vi "DAC_manual_ramp.vi"() -> ()   [LabVIEW 2013]
uses:
  <vilib>/DAQmx/read.llb/DAQmx Read (Analog 2D DBL NChan NSamp).vi
  <vilib>/DAQmx/create/channels.llb/DAQmx Create Channel (AI-Voltage-Basic).vi
  <vilib>/DAQmx/miscellaneous.llb/DAQmx Fill In Error Info.vi
  <resource>/objmgr/daqmx.rc
panel:
  out "Imin":dbl
  out "R":dbl
  in  "Back to\ninit value":bool
  in  "ADC Gain":u32(ring)=1 items=["1e6"=1000, "1e7"=100, "1e8"=10, "1e9"=1]
  in  "Save data":bool
  out "Ydata":dbl[][](array[numeric])
  out "Xdata":dbl[][](array[numeric])
  out "ADC values":dbl[](array[numeric])
  in  "DAC param":T1={"IP Adress FPGA"="192.168.137.11", "Delay(us)"=100, "Busses to use"=[TRUE, TRUE, TRUE, TRUE, TRUE, FALSE, FALSE, FALSE], "max"=0.5, "min"=-2.0}
  in  "Clear graph":bool
  in  "ADC channel":dbl
  in  "Stop":bool
  in  "Go":bool
  in  "time per pt (ms)":dbl=100.0
  in  "Xparam":dbl
  out "XY Graph":cluster{dbl[], dbl[]}(graph)
  in  "Nb of points":u32=101
  in  "Ramps":T2(array[cluster]) {"index" items=["0", "1", "2", "3", "4", "5", "6", "7"]; "bus" items=["0", "1", "2", "3", "4", "5", "6", "7"]}
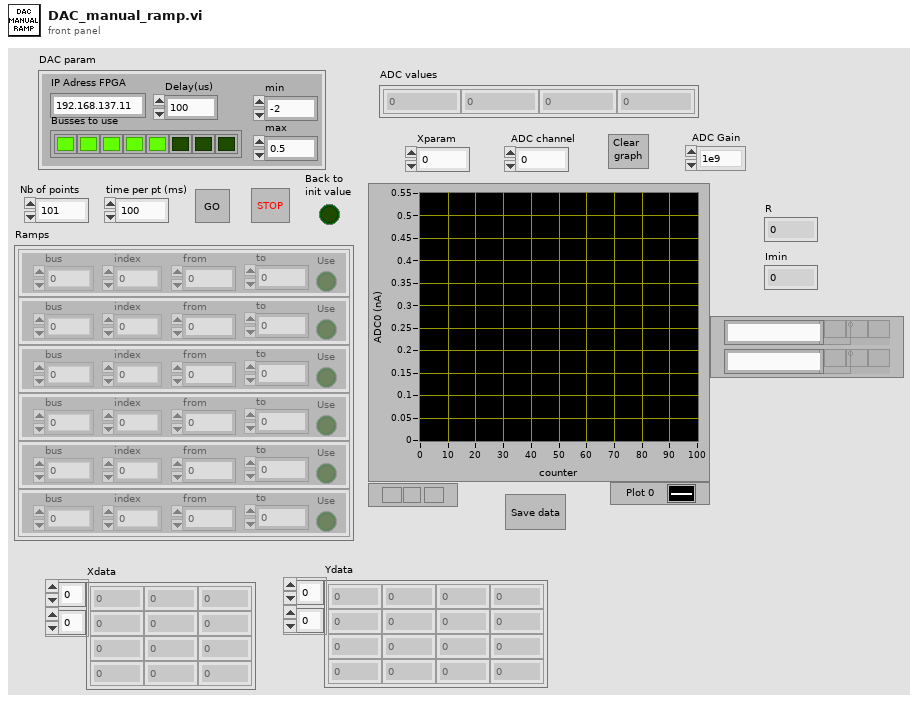
[diagram p1: front panel]
types:
  T1 = cluster{"IP Adress FPGA":string, "Delay(us)":u8, "Busses to use":bool[], "max":dbl, "min":dbl}
  T2 = cluster{"bus":u16, "index":u16, "from":dbl, "to":dbl, "Use":bool}[]
  T3 = enum8{"start movement", "buses to use", "delay", "value", "stop", ""}
  T4 = cluster{"bus":u16, "index":u16, "from":dbl, "to":dbl, "Use":bool}
  T5 = typedef "fpga-bitfile-ref.ctl" = refnum<k20>
  T6 = enum8{"start movement", "buses to use", "delay", "value"}
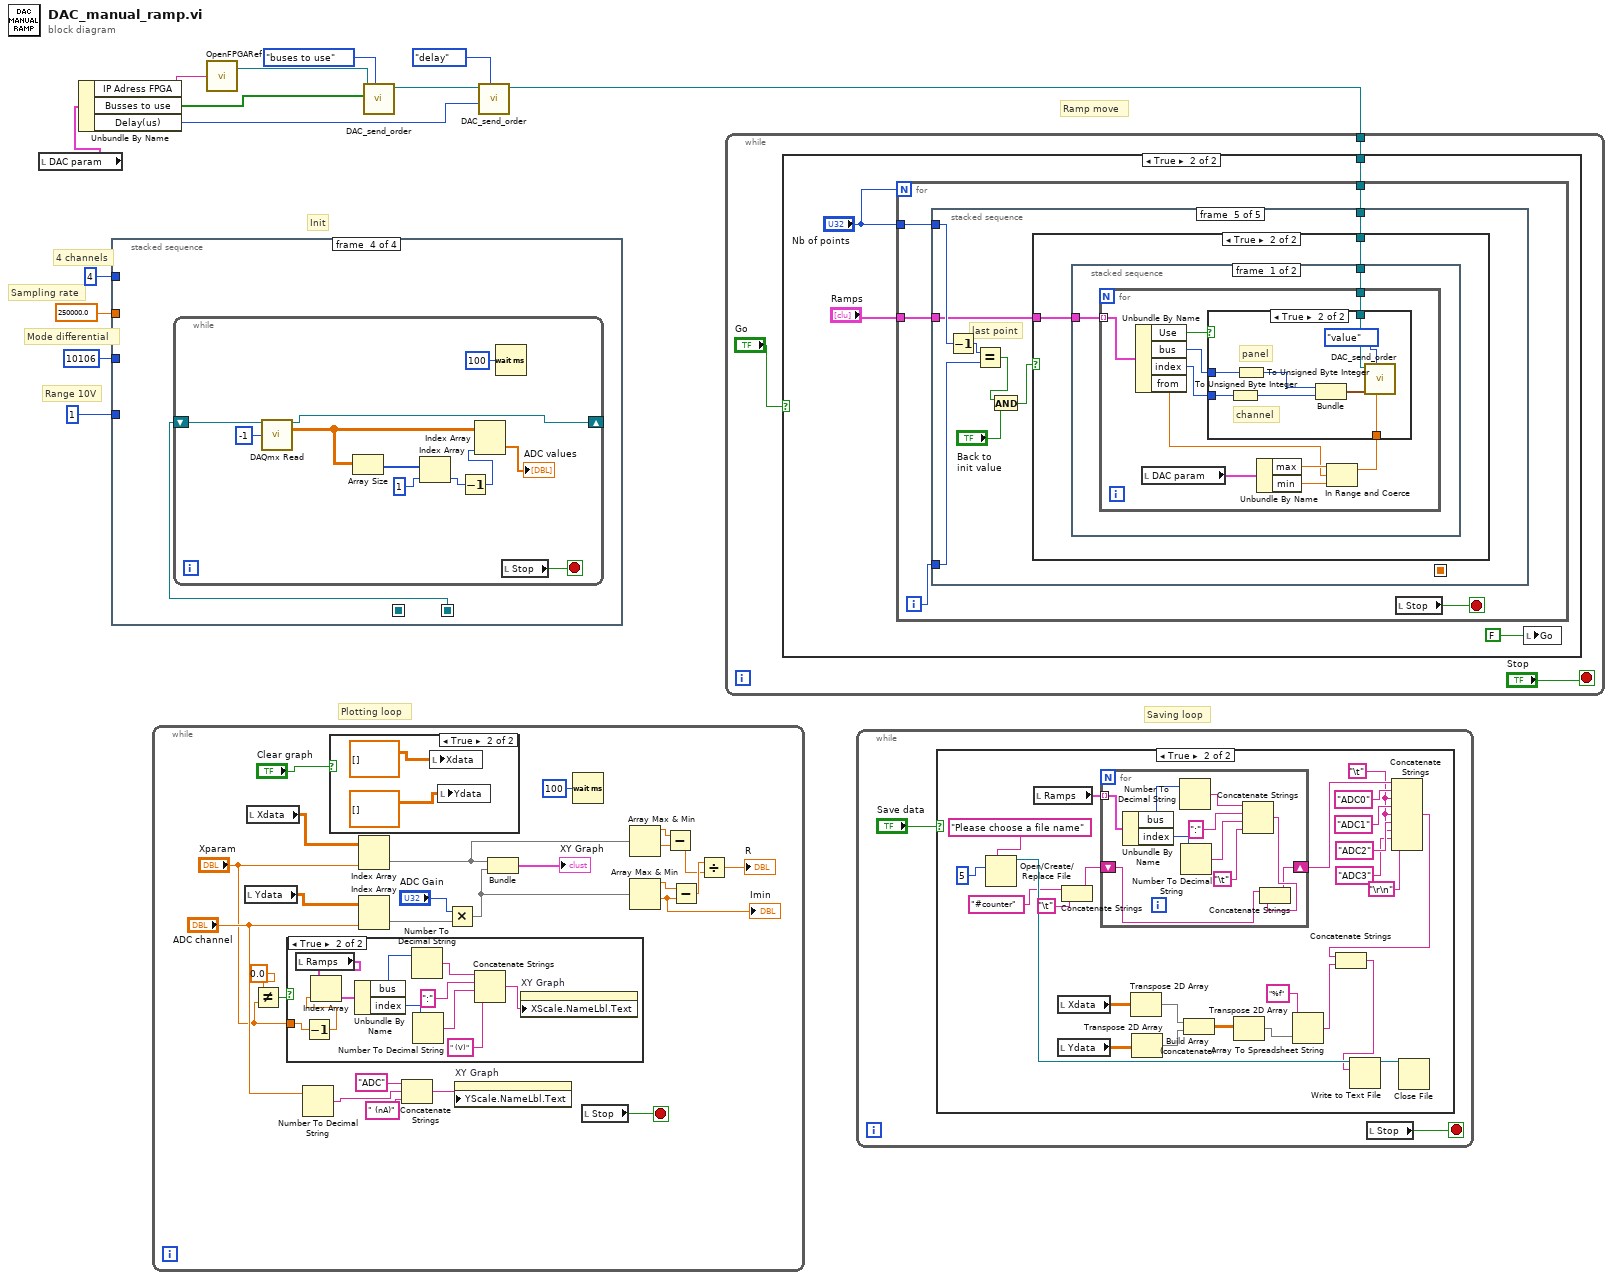
[diagram p0: block diagram]
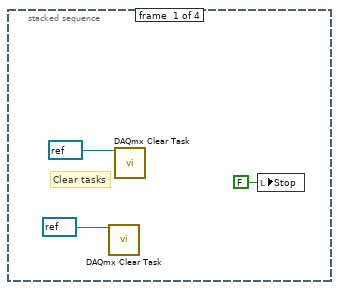
[diagram p2: hidden frame]
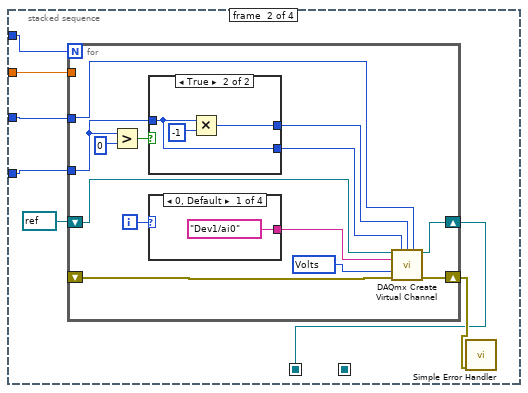
[diagram p3: hidden frame]
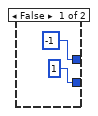
[diagram p4: hidden frame]
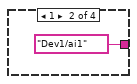
[diagram p5: hidden frame]
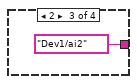
[diagram p6: hidden frame]
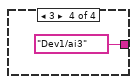
[diagram p7: hidden frame]
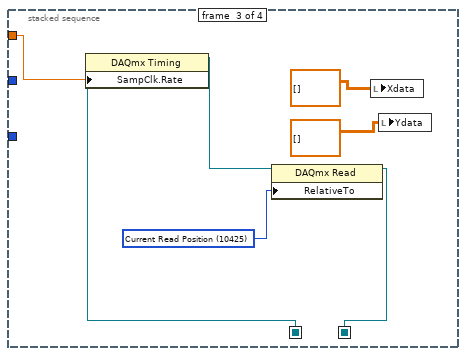
[diagram p8: hidden frame]
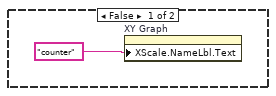
[diagram p10: hidden frame]
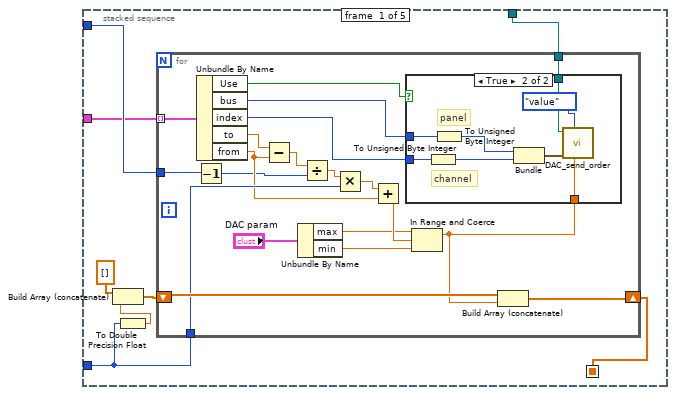
[diagram p12: hidden frame]
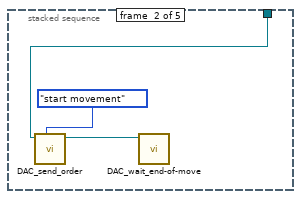
[diagram p14: hidden frame]
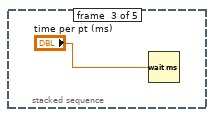
[diagram p15: hidden frame]
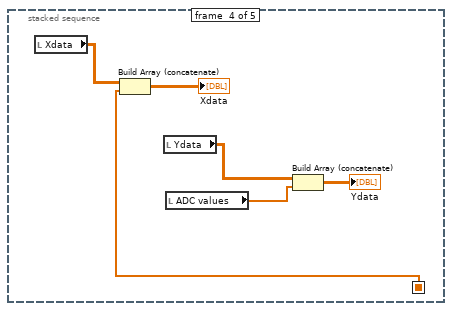
[diagram p16: hidden frame]
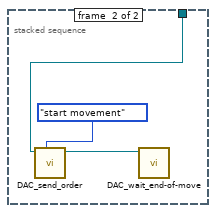
[diagram p19: hidden frame]
diagram:
  # "Init"
  # "Sampling rate"
  # "Mode differential"
  # "Range 10V"
  # "4 channels"
  # "Plotting loop"
  # "Ramp move"
  # "Saving loop"
  n1 = local read "DAC param"() -> (w6:T1)
  n2 = Unbundle By Name(w6) -> ("IP Adress FPGA"=w9:string, "Busses to use"=w8:bool[], "Delay(us)"=w7:u8)
  n3 = stacked-sequence {
    seq-local: [_ w17 _ _] -> [_ _ w51 _]
    seq-local: [_ _ w48 _] -> [_ _ _ w53]
    tunnel: 4 -> [_ w22 _ _]
    tunnel: 10106 -> [_ w21 _ _]
    tunnel: 1 -> [_ w20 _ _]
    tunnel: 250000.0 -> [_ w19 w52 _]
    frame #0 {
      # "Clear tasks"
      n4 = call <vilib>:"DAQmx Clear Task.vi"("task in"=refnum<k21> refnum ("task out in")) -> ()  [unwired: 14 in, 1 out]
      n5 = call <vilib>:"DAQmx Clear Task.vi"("task in"=refnum<k21> refnum ("task out in")) -> ()  [unwired: 14 in, 1 out]
      n6 = local write "Stop"(FALSE ("Stop")) -> ()
    }
    frame #1 {
      n7 = for {
        N: w22 -> [_]
        shift-right: [w24] -> w17
        shift-left: refnum<k21> refnum ("task out") -> [w36]
        shift-right: [w33] -> w23
        shift-left: _ -> [w25]
        tunnel: w20 -> [w30]
        tunnel: w21 -> [w26]
        tunnel: w19 -> [_]
        i -> [w27]
        w34 = 10348 items=["Volts"=10348, "From Custom Scale"=10065] ("units")
        n8 = Greater?(x=w30, y=i16 0) -> (0:w31:bool)
        n9 = case shown="True" w31 {
          tunnel: w30 -> [_ w39]
          tunnel: [i16 -1 w40] -> w32
          tunnel: [i16 1 ("Range") w39] -> w28
          frame False {
          }
          frame True {
            n10 = Multiply(x=w39, y=i16 -1) -> (x*y=w40:i32)
          }
        }
        n11 = case shown="0, Default" w27 {
          tunnel: [tag "Dev1/ai0" ("physical channels") tag "Dev1/ai1" ("physical channels") tag "Dev1/ai2" ("physical channels") tag "Dev1/ai3" ("physical channels")] -> w35
          frame 0, Default {
          }
          frame 1 {
          }
          frame 2 {
          }
          frame 3 {
          }
        }
        n12 = call-poly <vilib>:"DAQmx Create Virtual Channel.vi"("task in"=w36, "maximum value"=w28, "minimum value"=w32, "input terminal configuration"=w26, "physical channels"=w35, "units"=w34, "error in"=w25) -> ("task out"=w24:refnum<k21>, "error out"=w33:errorcluster)  [unwired: 2 in, 5 out]
      }
      n13 = call <vilib>:"Simple Error Handler.vi"("error in (no error)"=w23) -> ()  [unwired: 4 in, 5 out]
    }
    frame #2 {
      w50 = 10425 items=["First Sample"=10424, "Current Read Position"=10425, "Reference Trigger"=10426, "First Pretrigger Sample"=10427, "Most Recent Sample"=10428] ("RelativeTo")
      n14 = property class="DAQmx Timing"(reference=w51, "SampClk.Rate"=w52) -> (reference out=w49:refnum<k21>)  [unwired: 1 in, 1 out]
      n15 = property class="DAQmx Read"(reference=w49, "RelativeTo"=w50) -> (reference out=w48:refnum<k21>)  [unwired: 1 in, 1 out]
      n16 = local write "Xdata"(dbl[][] []) -> ()
      n17 = local write "Ydata"(dbl[][] []) -> ()
    }
    frame #3 {
      n18 = while {
        shift-right: [w58] -> _
        shift-left: w53 -> [w59]
        stop <- w64 stop-if-true
        n19 = call-poly <vilib>:"DAQmx Read.vi"("task/channels in"=w59, "number of samples per channel"=-1) -> ("task out"=w58:refnum<k21>, "data"=w61:dbl[][])  [unwired: 11 in, 1 out]
        n20 = Array Size(array=w61) -> (size(s)=w62:i32[])
        n21 = Index Array(array=w62, index=1) -> (element=w56:i32)
        n22 = Decrement(x=w56) -> (x-1=w55:i32)
        n23 = Index Array(array=w61, index (col)=w55) -> (element=→"ADC values":dbl[])  [unwired: 1 in]
        n24 = Wait (ms)(milliseconds to wait=100) -> ()  [unwired: 1 out]
        n25 = local read "Stop"() -> (w64:bool)
      }
    }
  }
  n26 = while {
    stop <- w89 stop-if-true
    n27 = local read "Ydata"() -> (w87:dbl[][])
    n28 = local read "Xdata"() -> (w88:dbl[][])
    n29 = Not Equal?(x=0.0, y="Xparam") -> (x != y?=w79:bool)
    n30 = case shown="True" w79 {
      tunnel: "Xparam" -> [_ w94]
      frame False {
        n31 = property on="XY Graph" class="XYGraph (strict)"("XScale.NameLbl.Text"="counter") -> ()  [unwired: 2 in, 2 out]
      }
      frame True {
        n32 = local read "Ramps"() -> (w103:T2)
        n33 = Decrement(x=w94) -> (x-1=w93:dbl)
        n34 = Index Array(array=w103, index=w93) -> (element=w102:T4)
        n35 = Unbundle By Name(w102) -> ("bus"=w101:u16, "index"=w100:u16)
        n36 = Number To Decimal String(number=w101) -> (decimal integer string=w98:string)  [unwired: 1 in]
        n37 = Number To Decimal String(number=w100) -> (decimal integer string=w99:string)  [unwired: 1 in]
        n38 = Concatenate Strings(w98, ":", w99, " (V)") -> (w95:string)
        n39 = property on="XY Graph" class="XYGraph (strict)"("XScale.NameLbl.Text"=w95) -> ()  [unwired: 2 in, 2 out]
      }
    }
    n40 = Number To Decimal String(number="ADC channel") -> (decimal integer string=w81:string)  [unwired: 1 in]
    n41 = case shown="True" "Clear graph" {
      frame False {
      }
      frame True {
        n42 = local write "Xdata"(dbl[][] []) -> ()
        n43 = local write "Ydata"(dbl[][] []) -> ()
      }
    }
    n44 = Index Array(array=w88, index (col)="Xparam") -> (element=w75:dbl[])  [unwired: 1 in]
    n45 = Index Array(array=w87, index (col)="ADC channel") -> (element=w71:dbl[])  [unwired: 1 in]
    n46 = Concatenate Strings("ADC", w81, " (nA)") -> (w82:string)
    n47 = Multiply(x="ADC Gain", y=w71) -> (x*y=w66:dbl[])
    n48 = property on="XY Graph" class="XYGraph (strict)"("YScale.NameLbl.Text"=w82) -> ()  [unwired: 2 in, 2 out]
    n49 = Bundle("Xdata"=w75, w66) -> (→"XY Graph":cluster{"Xdata":dbl[], dbl[]})  [unwired: 1 in]
    n50 = Wait (ms)(milliseconds to wait=100) -> ()  [unwired: 1 out]
    n51 = local read "Stop"() -> (w89:bool)
    n52 = Array Max & Min(array=w75) -> (max value=w74:dbl, min value=w73:dbl)  [unwired: 2 out]
    n53 = Array Max & Min(array=w66) -> (max value=w72:dbl, min value=w65:dbl)  [unwired: 2 out]
    "Imin" <- w65
    n54 = Subtract(x=w74, y=w73) -> (x-y=w68:dbl)
    n55 = Subtract(x=w72, y=w65) -> (x-y=w69:dbl)
    n56 = Divide(x=w69, y=w68) -> (x/y=→"R":dbl)
  }
  n57 = call "OpenFPGARef.vi"("IP Address"=w9) -> ("FPGA VI Reference Out"=w10:T5)  [unwired: 1 out]
  n58 = call "DAC_send_order.vi"("order"=T3."buses to use", "buses to use"=w8, "FPGA VI Reference In"=w10) -> ("FPGA VI Reference Out"=w11:T5)  [unwired: 8 in]
  n59 = call "DAC_send_order.vi"("order"=T3."delay", "delay between steps (us)"=w7, "FPGA VI Reference In"=w11) -> ("FPGA VI Reference Out"=w5:T5)  [unwired: 8 in]
  n60 = while {
    tunnel: w5 -> [w105]
    stop <- "Stop" stop-if-true
    n61 = case shown="True" "Go" {
      tunnel: w105 -> [_ w110]
      frame False {
      }
      frame True {
        n62 = for {
          N: "Nb of points" -> [_]
          tunnel: "Nb of points" -> [w115]
          tunnel: w110 -> [w114]
          tunnel: "Ramps" -> [w111]
          i -> [w113]
          stop <- w112 stop-if-true
          n63 = stacked-sequence {
            seq-local: [w121 _ _ _ _] -> [_ _ _ w161 _]
            tunnel: w115 -> [w123 _ _ _ w169]
            tunnel: w114 -> [w122 w154 _ _ w166]
            tunnel: w113 -> [w120 _ _ _ w165]
            tunnel: w111 -> [w116 _ _ _ w167]
            frame #0 {
              n64 = To Double Precision Float(number=w120) -> (double precision float=w118:dbl)
              n65 = Build Array (concatenate)(dbl[] [], w118) -> (w117:dbl[])
              n66 = for {
                tunnel: w116 -> [w138] mode=indexing
                tunnel: w123 -> [w143]
                tunnel: w122 -> [w142]
                shift-right: [w141] -> w121
                shift-left: w117 -> [w140]
                tunnel: w120 -> [w139]
                n67 = Decrement(x=w143) -> (x-1=w132:u32)
                n68 = Unbundle By Name(w138) -> ("Use"=w125:bool, "bus"=w131:u16, "index"=w130:u16, "to"=w137:dbl, "from"=w133:dbl)
                n69 = Subtract(x=w137, y=w133) -> (x-y=w136:dbl)
                n70 = Unbundle By Name("DAC param") -> ("max"=w126:dbl, "min"=w127:dbl)
                n71 = Divide(x=w136, y=w132) -> (x/y=w135:dbl)
                n72 = Multiply(x=w135, y=w139) -> (x*y=w134:dbl)
                n73 = Add(x=w134, y=w133) -> (x+y=w128:dbl)
                n74 = In Range and Coerce(upper limit=w126, x=w128, lower limit=w127) -> (coerced(x)=w124:dbl)  [unwired: 1 out]
                n75 = case shown="True" w125 {
                  tunnel: w142 -> [_ w151]
                  tunnel: w131 -> [_ w146]
                  tunnel: w130 -> [_ w145]
                  tunnel: w124 -> [_ w144]
                  frame False {
                  }
                  frame True {
                    # "channel"
                    # "panel"
                    n76 = To Unsigned Byte Integer(number=w145) -> (unsigned 8bit integer=w148:u8)
                    n77 = To Unsigned Byte Integer(number=w146) -> (unsigned 8bit integer=w149:u8)
                    n78 = Bundle(w149, w148) -> (w147:cluster{u8, u8})  [unwired: 1 in]
                    n79 = call "DAC_send_order.vi"("DAC goto value"=w144, "order"=T6."value", "Cluster"=w147, "FPGA VI Reference In"=w151) -> ()  [unwired: 3 in, 5 out]
                  }
                }
                n80 = Build Array (concatenate)(w140, w124) -> (w141:dbl[])
              }
            }
            frame #1 {
              n81 = call "DAC_send_order.vi"("order"=T6."start movement", "FPGA VI Reference In"=w154) -> ("FPGA VI Reference Out"=w152:T5)  [unwired: 5 in, 4 out]
              n82 = call "DAC_wait_end-of-move.vi"("FPGA VI Reference In"=w152) -> ()  [unwired: 10 in, 1 out]
            }
            frame #2 {
              n83 = Wait (ms)(milliseconds to wait="time per pt (ms)") -> ()  [unwired: 1 out]
            }
            frame #3 {
              n84 = local read "Xdata"() -> (w158:dbl[][])
              n85 = Build Array (concatenate)(w158, w161) -> (→"Xdata":dbl[][])
              n86 = local read "Ydata"() -> (w157:dbl[][])
              n87 = local read "ADC values"() -> (w156:dbl[])
              n88 = Build Array (concatenate)(w157, w156) -> (→"Ydata":dbl[][])
            }
            frame #4 {
              # "last point"
              n89 = Decrement(x=w169) -> (x-1=w168:u32)
              n90 = Equal?(x=w168, y=w165) -> (x = y?=w162:bool)
              n91 = And(x=w162, y="Back to\ninit value") -> (x .and. y?=w163:bool)
              n92 = case shown="True" w163 {
                tunnel: w167 -> [_ w171]
                tunnel: w166 -> [_ w170]
                frame False {
                }
                frame True {
                  n93 = stacked-sequence {
                    tunnel: w171 -> [w173 _]
                    tunnel: w170 -> [w172 w192]
                    frame #0 {
                      n94 = for {
                        tunnel: w173 -> [w183] mode=indexing
                        tunnel: w172 -> [w179]
                        n95 = Unbundle By Name(w183) -> ("Use"=w182:bool, "bus"=w181:u16, "index"=w180:u16, "from"=w175:dbl)
                        n96 = local read "DAC param"() -> (w178:T1)
                        n97 = Unbundle By Name(w178) -> ("max"=w176:dbl, "min"=w177:dbl)
                        n98 = In Range and Coerce(upper limit=w176, x=w175, lower limit=w177) -> (coerced(x)=w174:dbl)  [unwired: 1 out]
                        n99 = case shown="True" w182 {
                          tunnel: w179 -> [_ w191]
                          tunnel: w181 -> [_ w186]
                          tunnel: w180 -> [_ w185]
                          tunnel: w174 -> [_ w184]
                          frame False {
                          }
                          frame True {
                            # "channel"
                            # "panel"
                            n100 = To Unsigned Byte Integer(number=w185) -> (unsigned 8bit integer=w188:u8)
                            n101 = To Unsigned Byte Integer(number=w186) -> (unsigned 8bit integer=w189:u8)
                            n102 = Bundle(w189, w188) -> (w187:cluster{u8, u8})  [unwired: 1 in]
                            n103 = call "DAC_send_order.vi"("DAC goto value"=w184, "order"=T6."value", "Cluster"=w187, "FPGA VI Reference In"=w191) -> ()  [unwired: 3 in, 5 out]
                          }
                        }
                      }
                    }
                    frame #1 {
                      n104 = call "DAC_send_order.vi"("order"=T6."start movement", "FPGA VI Reference In"=w192) -> ("FPGA VI Reference Out"=w193:T5)  [unwired: 5 in, 4 out]
                      n105 = call "DAC_wait_end-of-move.vi"("FPGA VI Reference In"=w193) -> ()  [unwired: 10 in, 1 out]
                    }
                  }
                }
              }
            }
          }
          n106 = local read "Stop"() -> (w112:bool)
        }
        n107 = local write "Go"(FALSE) -> ()
      }
    }
  }
  n108 = while {
    stop <- w195 stop-if-true
    n109 = case shown="True" "Save data" {
      frame False {
      }
      frame True {
        w205 = "\t"
        n110 = Open/Create/Replace File(prompt="Please choose a file name", operation (0:open)=5) -> (refnum out=w204:refnum<file>)  [unwired: 4 in, 2 out]
        n111 = local read "Ramps"() -> (w212:T2)
        n112 = local read "Xdata"() -> (w219:dbl[][])
        n113 = local read "Ydata"() -> (w218:dbl[][])
        n114 = Concatenate Strings("#counter", "\t") -> (w198:string)
        n115 = for {
          tunnel: w212 -> [w226] mode=indexing
          shift-right: [w223] -> w211
          shift-left: w198 -> [w225]
          n116 = Unbundle By Name(w226) -> ("bus"=w227:u16, "index"=w228:u16)
          n117 = Number To Decimal String(number=w227) -> (decimal integer string=w230:string)  [unwired: 1 in]
          n118 = Number To Decimal String(number=w228) -> (decimal integer string=w229:string)  [unwired: 1 in]
          n119 = Concatenate Strings(w230, ":", w229, "\t") -> (w224:string)
          n120 = Concatenate Strings(w225, w224) -> (w223:string)
        }
        n121 = Transpose 2D Array(2D array=w219) -> (transposed array=w217:dbl[][])
        n122 = Transpose 2D Array(2D array=w218) -> (transposed array=w216:dbl[][])
        n123 = Build Array (concatenate)(w217, w216) -> (w215:dbl[][])
        n124 = Transpose 2D Array(2D array=w215) -> (transposed array=w214:dbl[][])
        n125 = Array To Spreadsheet String(array=w214, 3:"%f") -> (spreadsheet string=w202:string)  [unwired: 1 in]
        n126 = Concatenate Strings(w211, "ADC0", w205, "ADC1", w205, "ADC2", w205, "ADC3", "\r\n") -> (w203:string)
        n127 = Concatenate Strings(w203, w202) -> (w201:string)
        n128 = Write to Text File(file (use dialog)=w204, text=w201) -> (refnum out=w197:refnum<file>)  [unwired: 2 in, 2 out]
        n129 = Close File(refnum=w197) -> ()  [unwired: 1 in, 2 out]
      }
    }
    n130 = local read "Stop"() -> (w195:bool)
  }
